vi "Check Channel Array Size.vi"(8 "error in":errorcluster, 10 "channel array size":i32, 11 "module in":refnum<class "Module.lvclass">) -> (0 "error out":errorcluster, 3 "module out":refnum<class "Module.lvclass">)   [LabVIEW 2017, in "Scan Engine Scripting.lvlib" / "Module.lvclass"]
uses:
  Module.lvclass
  Scan Engine Custom Device.lvlib
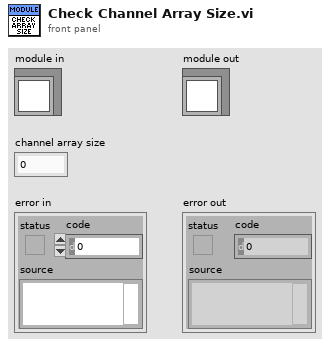
[diagram p1: front panel]
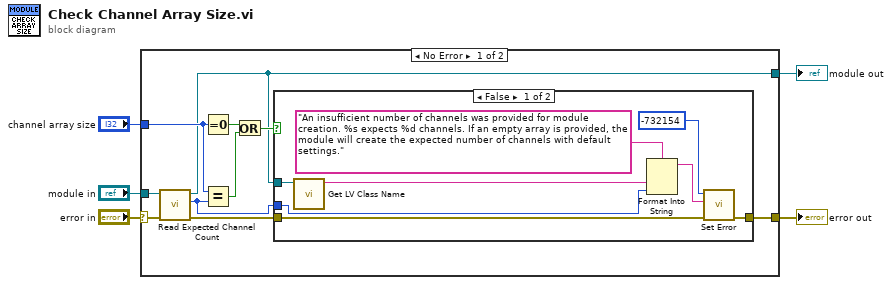
[diagram p0: block diagram]
diagram:
  n1 = case shown="No Error" "error in" {
    selector: "error in" -> [w14 w26]
    tunnel: [w8 w26] -> w4
    tunnel: [w7 w25] -> w2
    tunnel: "module in" -> [w15 w25]
    tunnel: "channel array size" -> [w13 _]
    frame No Error {
      n2 = call-dynamic "Read Expected Channel Count.vi"("error in"=w14, "module in"=w15) -> ("error out"=w9:errorcluster, "expected channel count"=w6:i32, "module out"=w7:refnum<class "Module.lvclass">)  [unwired: 7 in]
      n3 = Equal To 0?(x=w13) -> (x = 0?=w12:bool)
      n4 = Equal?(x=w13, y=w6) -> (x = y?=w11:bool)
      n5 = Or(x=w12, y=w11) -> (x .or. y?=w10:bool)
      n6 = case shown="False" w10 {
        tunnel: w9 -> [w21 w24]
        tunnel: [w22 w24] -> w8
        tunnel: w7 -> [w18 _]
        tunnel: w6 -> [w16 _]
        frame False {
          n7 = call <vilib>:"Get LV Class Name.vi"("object"=w18) -> ("class name"=w17:string)  [unwired: 9 in, 1 out]
          n8 = Format Into String(format string="An insufficient number of channels was provided for module creation. %s expects %d channels. If an empty array is provided, the module will create the expected number of channels with default settings.", w17, w16) -> (resulting string=w20:string)  [unwired: 2 in, 1 out]
          n9 = call "Set Error.vi"("error in (no error)"=w21, "Message"=w20, "Code"=-732154) -> ("error out"=w22:errorcluster)  [unwired: 8 in]
        }
        frame True {
        }
      }
    }
    frame Error {
    }
  }
  "error out" <- w4
  "module out" <- w2
